vi "RTMain (1).vi"   [LabVIEW 2017]
doc: "Main VI to be run from cRIO controller. Can be started before or after the HostMain.vi on host computer."
uses:
  RTControl/StopGLOBAL.vi
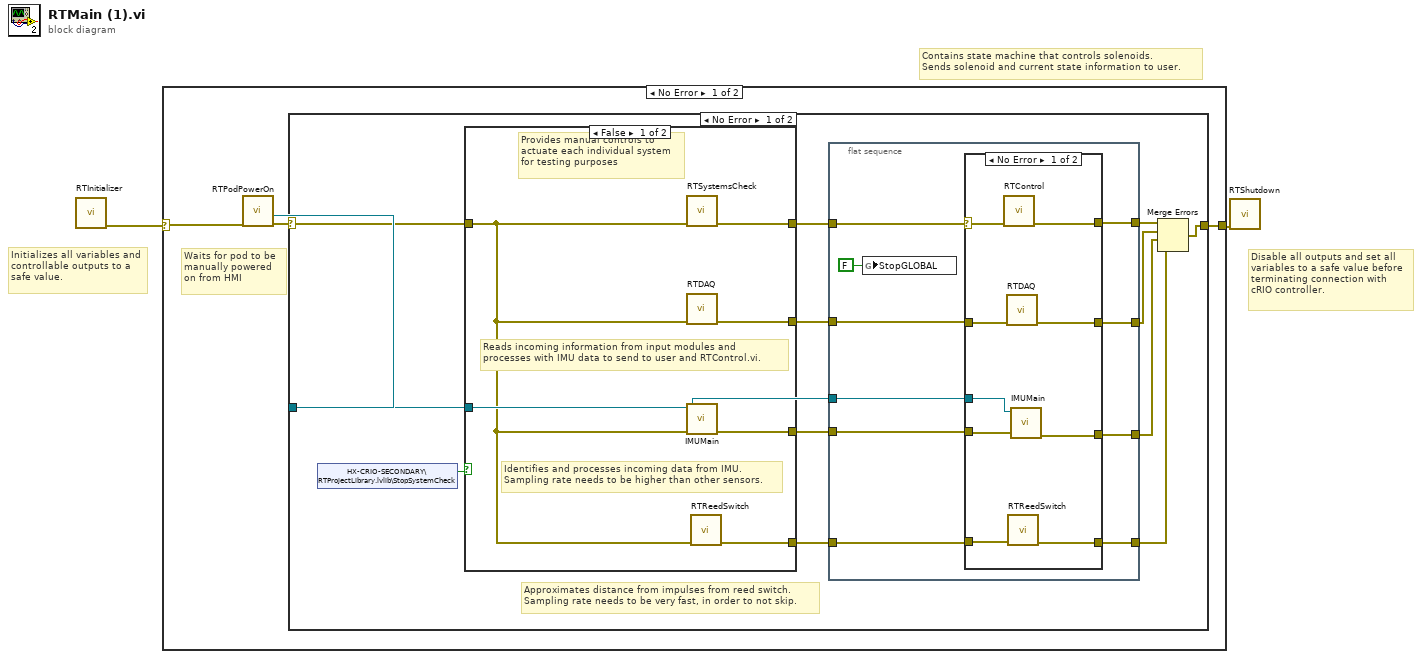
[diagram p0: block diagram]
diagram:
  # "Contains state machine that controls solenoids.\nSends solenoid and current state information to user."
  # "Disable all outputs and set all\nvariables to a safe value before\nterminating connection with \ncRIO controller."
  # "Initializes all variables and\ncontrollable outputs to a \nsafe value."
  n1 = call "RTInitializer.vi"() -> ("error out"=w1:errorcluster)  [unwired: 11 in]
  n2 = case shown="No Error" w1 {
    selector: w1 -> [w6 w50]
    tunnel: [w5 w50] -> w2
    frame No Error {
      # "Waits for pod to be\nmanually powered\non from HMI"
      n3 = call "RTPodPowerOn.vi"("error in (no error)"=w6) -> ("error out"=w4:errorcluster, "VISA Refnum out"=w3:refnum<visa-resource-name>)  [unwired: 9 in]
      n4 = case shown="No Error" w4 {
        selector: w4 -> [w15 w49]
        tunnel: [w18 w49] -> w5
        tunnel: w3 -> [w8 _]
        frame No Error {
          # "Approximates distance from impulses from reed switch.\nSampling rate needs to be very fast, in order to not skip."
          n5 = shared-variable "HX-CRIO-SECONDARY\\RTProjectLibrary.lvlib\\StopSystemCheck"() -> (w7:bool)  [unwired: 1 in, 1 out]
          n6 = case shown="False" w7 {
            tunnel: [w24 w25] -> w16
            tunnel: w15 -> [w23 w25]
            tunnel: [w22 w25] -> w14
            tunnel: [w21 w25] -> w13
            tunnel: [w20 w25] -> w12
            tunnel: w8 -> [w19 _]
            frame False {
              # "Reads incoming information from input modules and\nprocesses with IMU data to send to user and RTControl.vi."
              # "Provides manual controls to\nactuate each individual system\nfor testing purposes"
              # "Identifies and processes incoming data from IMU.\nSampling rate needs to be higher than other sensors."
              n7 = call "RTSystemsCheck.vi"("error in"=w23) -> ("error out"=w24:errorcluster)  [unwired: 10 in]
              n8 = call "RTDAQ.vi"("error in (no error)"=w23) -> ("error out"=w21:errorcluster)  [unwired: 10 in]
              n9 = call "IMUMain.vi"("error in"=w23, "VISA Refnum out"=w19) -> ("error out"=w20:errorcluster)  [unwired: 9 in]
              n10 = call "RTReedSwitch.vi"("error in (no error)"=w23) -> ("error out"=w22:errorcluster)  [unwired: 10 in]
            }
            frame True {
            }
          }
          n11 = flat-sequence {
            tunnel: [w35] -> w17
            tunnel: w16 -> [w34]
            tunnel: w14 -> [w33]
            tunnel: w13 -> [w32]
            tunnel: w12 -> [w31]
            tunnel: [w30] -> w11
            tunnel: [w29] -> w10
            tunnel: [w28] -> w9
            tunnel: w8 -> [w27]
            frame #0 {
              n12 = global write "StopGLOBAL.vi" "StopGLOBAL"(FALSE ("StopGLOBAL")) -> ()
              n13 = case shown="No Error" w34 {
                selector: w34 -> [w43 w48]
                tunnel: [w44 w48] -> w35
                tunnel: w33 -> [w42 w45]
                tunnel: w32 -> [w41 w47]
                tunnel: w31 -> [w40 w46]
                tunnel: [w39 w45] -> w30
                tunnel: [w38 w47] -> w29
                tunnel: [w37 w46] -> w28
                tunnel: w27 -> [w36 _]
                frame No Error {
                  n14 = call "RTControl.vi"("error in (no error)"=w43) -> ("error out"=w44:errorcluster)  [unwired: 10 in]
                  n15 = call "RTDAQ.vi"("error in (no error)"=w41) -> ("error out"=w38:errorcluster)  [unwired: 10 in]
                  n16 = call "RTReedSwitch.vi"("error in (no error)"=w42) -> ("error out"=w39:errorcluster)  [unwired: 10 in]
                  n17 = call "IMUMain.vi"("error in"=w40, "VISA Refnum out"=w36) -> ("error out"=w37:errorcluster)  [unwired: 9 in]
                }
                frame Error {
                }
              }
            }
          }
          n18 = Merge Errors(w17, w10, w9, w11) -> (w18:errorcluster)
        }
        frame Error {
        }
      }
    }
    frame Error {
    }
  }
  n19 = call "RTShutdown.vi"("error in"=w2) -> ()  [unwired: 10 in, 1 out]
